vi "Open.vi"(7 "I2C Channel (0)":u8, 8 "Error In":errorcluster, 9 "Resolution":enum16{"2g", "4g", "8g", "16g"}(ring), 10 "I2C Slave Address":T1, 11 "LINX Resource":T2) -> (0 "Error Out":errorcluster, 1 "Resolution":enum16{"2g", "4g", "8g", "16g"}(ring), 3 "LINX Resource":T2)   [LabVIEW 2014, in "LMH-LINX.lvlib" / "ADXL345.lvlib"]
doc: "Open the I2C master, initialize the ADXL345, set it's resolution and bring it out of sleep mode."
uses:
  ADXL345.lvlib
  Private/Type Defs/LINX Ref.ctl
  Private/Type Defs/Platform.ctl
  Private/Type Defs/Interface.ctl
  Private/Device/Type Defs/LINX Device Config.ctl
  Private/Device/Type Defs/TCP Config.ctl
  Private/Device/Type Defs/Channels.ctl
  Address.ctl
  Private/Local IO/LinxI2cWrite.vi
  Utilities/Check Channel.vi
  Private/Utilties/Generate Error.vi
  LMH-LINX.lvlib
  Private/Device/Device.lvlib
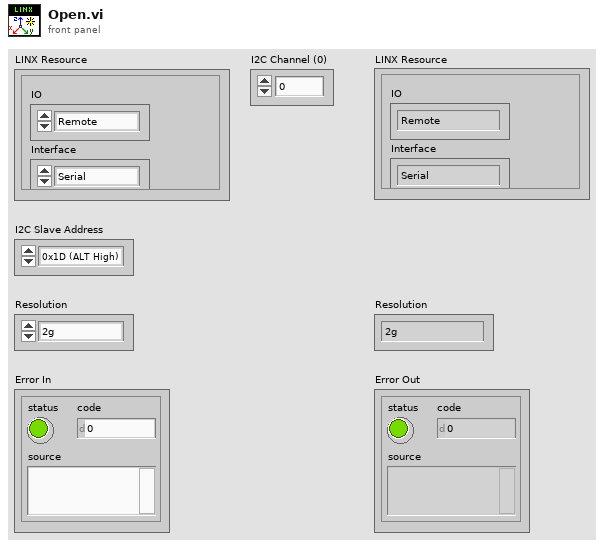
[diagram p1: front panel]
types:
  T1 = typedef "LMH-LINX.lvlib/ADXL345.lvlib/Address.ctl" = enum16{"0x1D (ALT High)", "0x53 (ALT Low)"}
  T2 = typedef "LMH-LINX.lvlib/LINX Ref.ctl" = cluster{"IO":T3, "Interface":T4, "LINX Device Config":T5}
  T3 = typedef "LMH-LINX.lvlib/Platform.ctl" = enum16{"Remote", "Local"}
  T4 = typedef "LMH-LINX.lvlib/Interface.ctl" = enum16{"Serial", "TCP"}
  T5 = typedef "LMH-LINX.lvlib/Device.lvlib/LINX Device Config.ctl" = cluster{"Interface":T4, "COM Port":refnum<visa-resource-name>, "TCP Configuration":T6, "Device Family":u8, "Device ID":u8, "Device Name":string, "TCP Ref":refnum<k5>, "Channels":T7}
  T6 = typedef "LMH-LINX.lvlib/Device.lvlib/TCP Config.ctl" = cluster{"IP Address":string, "Port":u16}
  T7 = typedef "LMH-LINX.lvlib/Channels.ctl" = cluster{"DI":u8[], "DO":u8[], "AI":u8[], "AO":u8[], "PWM":u8[], "QE":u8[], "UART":u8[], "I2C 2":u8[], "SPI":u8[], "CAN":u8[], "Servo":u8[], "AI Ref (V)":dbl, "AI Resolution (Bits)":u8, "AO Ref (V)":dbl, "AO Resolution (Bits)":u8}
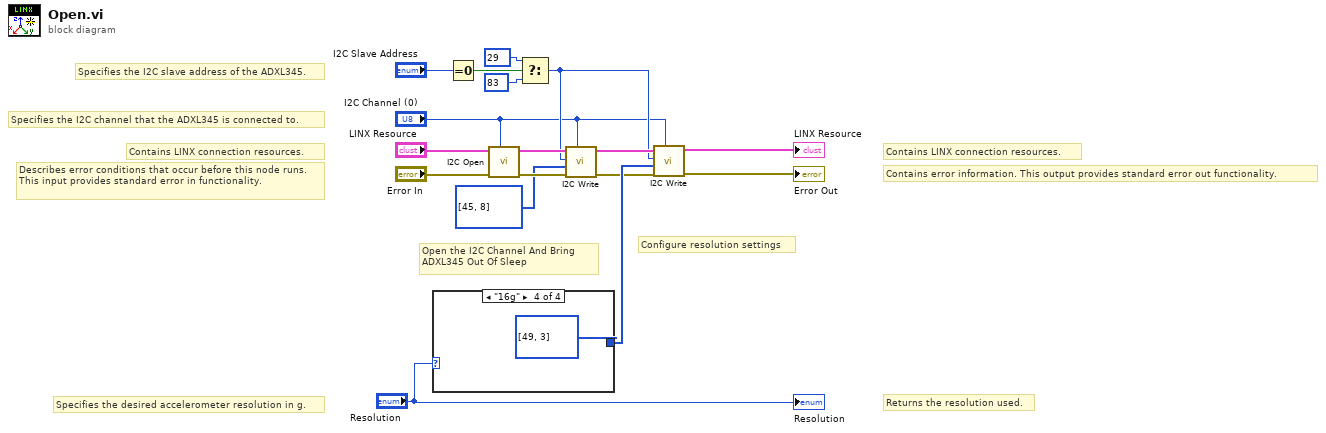
[diagram p0: block diagram]
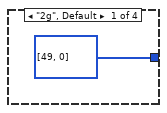
[diagram p2: hidden frame]
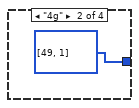
[diagram p3: hidden frame]
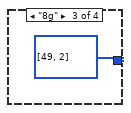
[diagram p4: hidden frame]
diagram:
  # "Specifies the I2C slave address of the ADXL345."
  # "Specifies the I2C channel that the ADXL345 is connected to."
  # "Specifies the desired accelerometer resolution in g."
  # "Returns the resolution used."
  # "Contains LINX connection resources."
  # "Contains error information. This output provides standard error out functionality."
  # "Contains LINX connection resources."
  # "Describes error conditions that occur before this node runs. This input provides standard error in functionality."
  # "Configure resolution settings"
  # "Open the I2C Channel And Bring \nADXL345 Out Of Sleep"
  n1 = case shown="\"16g\"" "Resolution" {
    tunnel: [u8[] [49, 0] ("Data") u8[] [49, 1] ("Data") u8[] [49, 2] ("Data") u8[] [49, 3] ("Data")] -> w7
    frame "2g", Default {
    }
    frame "4g" {
    }
    frame "8g" {
    }
    frame "16g" {
    }
  }
  n2 = Equal To 0?(x="I2C Slave Address") -> (x = 0?=w13:bool)
  n3 = call "I2C Open.vi"("I2C Channel (0)"="I2C Channel (0)", "Error In"="Error In", "LINX Resource"="LINX Resource") -> ("Error Out"=w16:errorcluster, "LINX Resource"=w17:T2)  [unwired: 7 in]
  n4 = Select(t=u8 29 ("I2C Slave Address (0)"), s=w13, f=u8 83 ("I2C Slave Address (0)")) -> (s? t:f=w2:u8)
  n5 = call "I2C Write.vi"("I2C Channel"="I2C Channel (0)", "Error In"=w16, "Data"=u8[] [45, 8], "I2C Slave Address (0)"=w2, "LINX Resource"=w17) -> ("Error Out"=w5:errorcluster, "LINX Resource"=w6:T2)  [unwired: 5 in]
  n6 = call "I2C Write.vi"("I2C Channel"="I2C Channel (0)", "Error In"=w5, "Data"=w7, "I2C Slave Address (0)"=w2, "LINX Resource"=w6) -> ("Error Out"=→"Error Out":errorcluster, "LINX Resource"=→"LINX Resource":T2)  [unwired: 5 in]
  "Resolution" <- "Resolution"
